vi "S Parameter Flatten Test Parameters.vi"(7 "Test Configuration (\"\")":string, 9 "error in (no error)":errorcluster, 10 "Parameter Variant":variant) -> (1 "error out":errorcluster, 2 "Parameter String":string)   [LabVIEW 2011]
uses:
  TypeDefs/SP Test Parameters.ctl
  TypeDefs/SP Stimulus Parameters.ctl
  TypeDefs/SP Frequency Units.ctl
  TypeDefs/SP Calibration State.ctl
  TypeDefs/SP Measurement.ctl
  TypeDefs/SP Parameters.ctl
  TypeDefs/SP Parameter.ctl
  TypeDefs/SP De-Embed.ctl
  TypeDefs/SP Adapter.ctl
  TypeDefs/SP Data.ctl
  TypeDefs/SP Display Parameters.ctl
  TypeDefs/SP Display Plot Controls Cluster.ctl
  TypeDefs/SP Marker Cluster.ctl
  TypeDefs/SP Marker Type.ctl
  TypeDefs/SP Display Trace Controls.ctl
  TypeDefs/SP Display Format.ctl
  TypeDefs/SP Display Data.ctl
  TypeDefs/SP Limit.ctl
  TypeDefs/SP Format.ctl
  TypeDefs/SP Limit Type.ctl
  TypeDefs/SP Limit Point.ctl
  Test Referential Limit.ctl
  TypeDefs/SP Filter.ctl
  TypeDefs/SP Filter Type.ctl
  TypeDefs/SP Filter Passband.ctl
  TypeDefs/SP Frequency Format.ctl
  TypeDefs/SP Filter Ripple.ctl
  TypeDefs/SP Attenuation Point.ctl
  TypeDefs/SP Attenuation Type.ctl
  TypeDefs/SP Skirt Rejection Point.ctl
  TypeDefs/SP Relative Loss.ctl
  S Parameter Version.vi
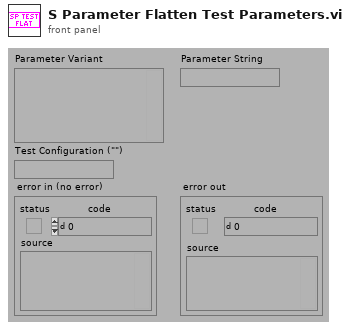
[diagram p1: front panel]
types:
  T1 = typedef "SP Test Parameters.ctl" = cluster{"Stimulus":T2, "Measurement":T5, "De-Embed":T8, "Display":T11, "Limits":T18[], "Filter Limits":T23[]}
  T2 = typedef "SP Stimulus Parameters.ctl" = cluster{"Use Instrument Settings":bool, "Blank Frequencies":bool, "Sweep Type":enum32{"Linear", "Logarithmic", "List", "Power", "CW"}, "Sweep":cluster{"Fstart":dbl, "Fstop":dbl, "Units":T3, "Points":i32}, "Power (dBm)":dbl, "IFBW (Hz)":dbl, "Sweep Time (s)":dbl, "Calibration":T4}
  T3 = typedef "SP Frequency Units.ctl" = enum16{"Hz", "kHz", "MHz", "GHz", "Points"}
  T4 = typedef "SP Calibration State.ctl" = cluster{"State":bool, "String":string}
  T5 = typedef "SP Measurement.ctl" = cluster{"Auto Select":bool, "Data Source":enum16{"VNA", "Data File"}, "Ports":i8, "Parameters":T6[]}
  T6 = typedef "SP Parameters.ctl" = cluster{"Channel":i8, "Parameter":T7}
  T7 = typedef "SP Parameter.ctl" = cluster{"Stimulus Port":i8, "Response Port":i8}
  T8 = typedef "SP De-Embed.ctl" = cluster{"De-Embed":bool, "Adapters":T9[]}
  T9 = typedef "SP Adapter.ctl" = cluster{"Port":i8, "Order":i8, "Model Number":string, "Serial Number":string, "SP Data":T10, "Run Type":enum16{"Most Recent", "Run #", "Match Field"}, "Run":i32, "Field":string, "Field Value":string}
  T10 = typedef "SP Data.ctl" = cluster{"F0":dbl, "dF":dbl, "Data":cdb[][]}
  T11 = typedef "SP Display Parameters.ctl" = cluster{"Lock Control":bool, "Retain Settings":bool, "Formatted Data":bool, "Plot Orientation":enum32{"Single", "Dual", "Quad"}, "Plot Controls":T12[]}
  T12 = typedef "SP Display Plot Controls Cluster.ctl" = cluster{"Trace Orientation":enum32{"Overlay", "Split"}, "Frequency":cluster{"Change Frequency":bool, "Start":dbl, "Stop":dbl, "Units":T3}, "Markers":T13[], "Traces":T15[]}
  T13 = typedef "SP Marker Cluster.ctl" = cluster{"Type":T14, "Frequency (MHz)":dbl}
  T14 = typedef "SP Marker Type.ctl" = enum16{"Frequency", "Trace Maximum", "Trace Minimum", "Limit Maximum", "Limit Minimum"}
  T15 = typedef "SP Display Trace Controls.ctl" = cluster{"Trace On":bool, "Measure":i32, "Format":T16, "Autoscale":bool, "Reference":dbl, "\nRefUnit":string, "Position":dbl, "Scale":dbl, "ScaleUnit":string, "LimitOn":bool, "LimitFill":bool, "Display Data":T17, "Show Markers":bool, "SXX":string}
  T16 = typedef "SP Display Format.ctl" = i32
  T17 = typedef "SP Display Data.ctl" = u16
  T18 = typedef "SP Limit.ctl" = cluster{"Parameter":T7, "Format":T19, "Limit Type":T20, "Points":T21[], "Referential Limit":T22, "Limit #":i8}
  T19 = typedef "SP Format.ctl" = enum16{"Log Mag", "Lin Mag", "SWR", "Phase", "Expanded Phase", "Delay", "Insertion Loss", "Isolation", "Return Loss"}
  T20 = typedef "SP Limit Type.ctl" = enum16{"Upper", "Lower", "Delta", "Filter", "Referential"}
  T21 = typedef "SP Limit Point.ctl" = cluster{"Frequency":dbl, "Value":dbl, "X":dbl, "Y":dbl, "Connected":bool}
  T22 = typedef "Test Referential Limit.ctl" = cluster{"Ref Limit":bool, "Ref Type":enum16{"Current", "Specify"}, "Model":string, "Serial":string, "Run Type":enum16{"Most Recent", "Run #", "Match Field"}, "Run":i32, "Field":string, "Field Value":string}
  T23 = typedef "SP Filter.ctl" = cluster{"Limit #":i8, "Parameter":T7, "Format":T19, "Filter Type":T24, "Passband":T25, "Ripple":T27, "Attenuation Points":T28[], "Skirt Points":T30[]}
  T24 = typedef "SP Filter Type.ctl" = enum16{"Lowpass", "Highpass", "Bandpass", "Bandstop"}
  T25 = typedef "SP Filter Passband.ctl" = cluster{"Start/Center":dbl, "Stop/Span":dbl, "Units":T3, "Freq Format":T26, "Bandwidth Attn":dbl, "Passband Limit":bool}
  T26 = typedef "SP Frequency Format.ctl" = enum16{"Start/Stop", "Center/Span"}
  T27 = typedef "SP Filter Ripple.ctl" = cluster{"Ripple Limit":bool, "Window On":bool, "Ripple":dbl, "Window":dbl, "Units":T3}
  T28 = typedef "SP Attenuation Point.ctl" = cluster{"Attenuation":dbl, "Type":T29, "Lower":dbl, "Upper":dbl, "Units":T3}
  T29 = typedef "SP Attenuation Type.ctl" = enum16{"Center", "Lower", "Upper"}
  T30 = typedef "SP Skirt Rejection Point.ctl" = cluster{"Relative":bool, "Connect":bool, "Frequency":dbl, "Units":T3, "Attenuation":dbl, "Relative Loss":T31, "Relative Freq":dbl}
  T31 = typedef "SP Relative Loss.ctl" = enum16{"Calculated Center", "Passband Minimum", "Passband Maximum", "Passband Average", "Frequency"}
  T32 = typedef "OGAB Version.ctl" = cluster{"Version":string, "Build Number":u32, "Build Date/Time":dbl}
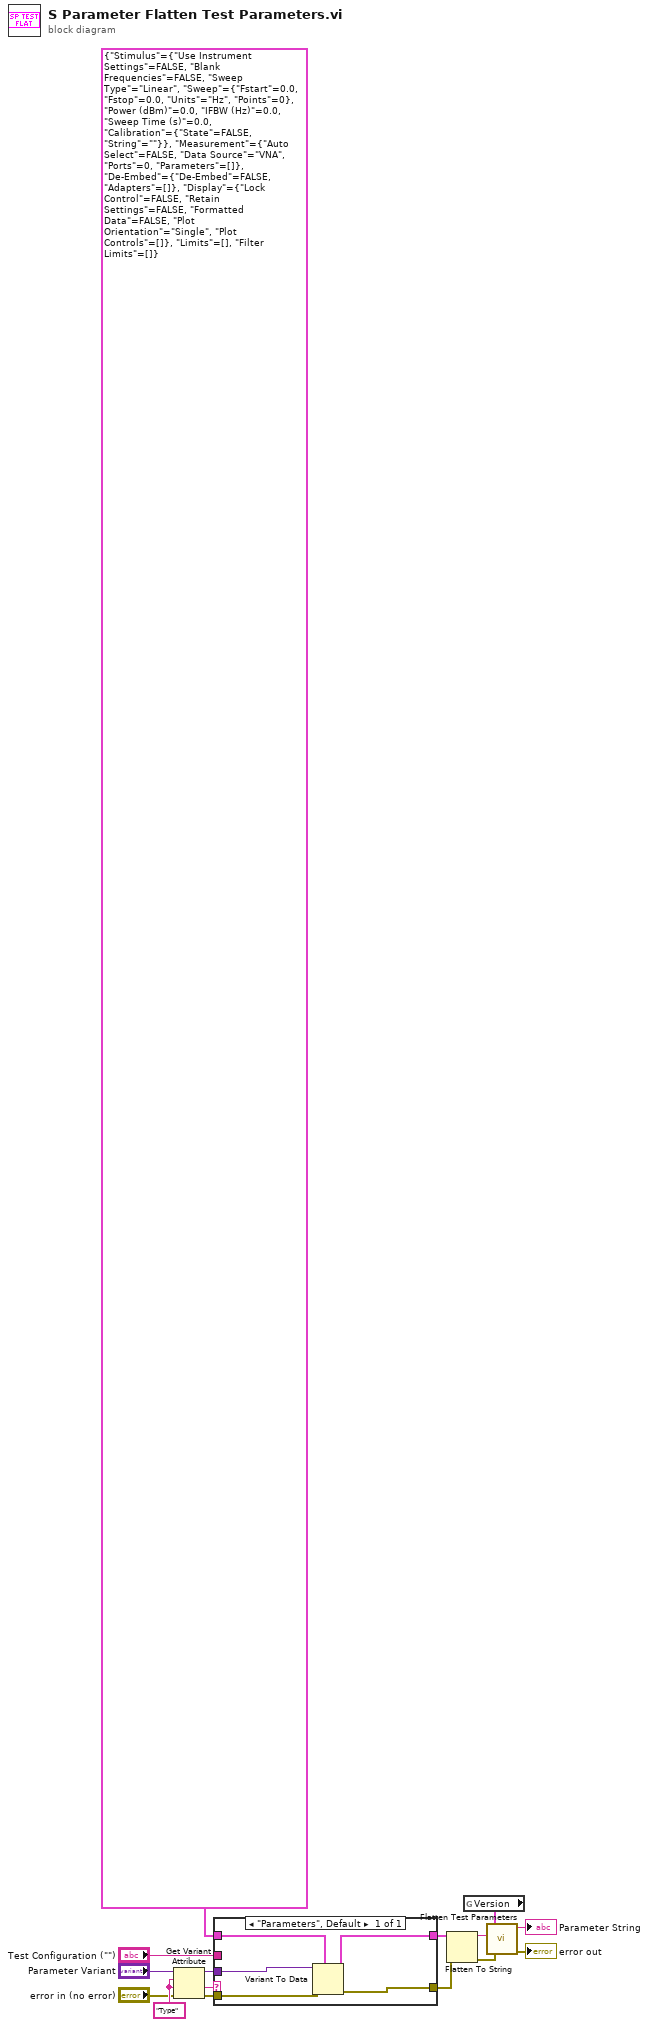
[diagram p0: block diagram]
diagram:
  w13 = "Type" ("name")
  n1 = Get Variant Attribute(Variant="Parameter Variant", name=w13, default value (empty Variant)=w13, error in="error in (no error)") -> (duplicate Variant=w14:variant, value=w12:string, error out=w5:errorcluster)  [unwired: 1 out]
  n2 = case shown="\"Parameters\", Default" w12 {
    tunnel: w14 -> [w20]
    tunnel: T1 {"Stimulus"={"Use Instrument Settings"=FALSE, "Blank Frequencies"=FALSE, "Sweep Type"=enum."Linear", "Sweep"={"Fstart"=0.0, "Fstop"=0.0, "Units"=enum."Hz", "Points"=0}, "Power (dBm)"=0.0, "IFBW (Hz)"=0.0, "Sweep Time (s)"=0.0, "Calibration"={"State"=FALSE, "String"=""}}, "Measurement"={"Auto Select"=FALSE, "Data Source"=enum."VNA", "Ports"=0, "Parameters"=[]}, "De-Embed"={"De-Embed"=FALSE, "Adapters"=[]}, "Display"={"Lock Control"=FALSE, "Retain Settings"=FALSE, "Formatted Data"=FALSE, "Plot Orientation"=enum."Single", "Plot Controls"=[]}, "Limits"=[], "Filter Limits"=[]} ("S Parameter Test Parameters") -> [w16]
    tunnel: [w17] -> w8
    tunnel: [w19] -> w6
    tunnel: w5 -> [w18]
    tunnel: "Test Configuration (\"\")" -> [_]
    frame "Parameters", Default {
      n3 = Variant To Data(error in=w18, type=w16, Variant=w20) -> (data=w17:T1, error out=w19:errorcluster)
    }
  }
  n4 = Flatten To String(anything=w8, error in (no error)=w6) -> (data string=w10:string, error out=w7:errorcluster)  [unwired: 3 out]
  n5 = global read "S Parameter Version.vi" "Version"() -> (w9:T32)
  n6 = call "Flatten Test Parameters.vi"("error in (no error)"=w7, "Flattened Test Parameters (\"\")"=w10, "Test Version"=w9) -> ("error out"=→"error out":errorcluster, "Flattened Test Parameters with Version"=→"Parameter String":string)  [unwired: 3 out]
